vi "XIPIN_Defective_Pixel_Correction_6_01_a.vi"   [LabVIEW 2017]
doc: "The Xilinx Defective Pixel Correction LogiCORE is a dynamic solution to remove defective pixels from a camera sensor array.\n------------------------------------\n<b>Need License</b> : Yes\n<b>Interface</b> : AXI4-Stream AXI4-Lite"
uses:
  <vilib>/rvi/XilinxIP/XIPIN_XNode/niFpgaXIPIN.xnode
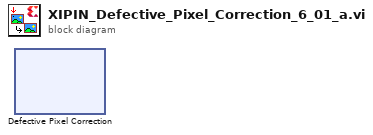
[diagram p0: block diagram]
diagram:
  n1 = xnode ("Defective Pixel Correction")() -> ()
